vi "Delete Service.vi"(8 "error in (no error)":errorcluster, 10 "Service Name":string[][](array[string]), 11 "Manejo Turnos in":refnum<class "Manejo Turnos.lvclass">) -> (0 "error out":errorcluster, 3 "Manejo Turnos out":refnum<class "Manejo Turnos.lvclass">)   [LabVIEW 2020, in "Manejo Turnos.lvlib" / "Manejo Turnos.lvclass"]
uses:
  Manejo Turnos.lvclass
  C:/Program Files (x86)/National Instruments/LabVIEW 2020/vi.lib/ActorFramework/Actor/Actor.lvclass
  <vilib>/ActorFramework/Actor/Actor.lvclass/Actor.ctl
  <vilib>/ActorFramework/Message Enqueuer/Message Enqueuer.lvclass/Message Enqueuer.ctl
  Manejo Turnos.lvclass/Manejo Turnos.ctl
  <vilib>/ActorFramework/Message Enqueuer/Init from Existing Queue.vi
  <vilib>/ActorFramework/Message Enqueuer/Enqueue.vi
  Manejo Turnos Messages/Delete Services Table Msg/Delete Services Table Msg.lvclass
  C:/Program Files (x86)/National Instruments/LabVIEW 2020/vi.lib/ActorFramework/Message/Message.lvclass
  <vilib>/ActorFramework/Message Priority Queue/Priority Enqueue.vi
  <vilib>/ActorFramework/Message Enqueuer/Message Enqueuer.lvclass
  <vilib>/ActorFramework/Actor/Actor.lvclass
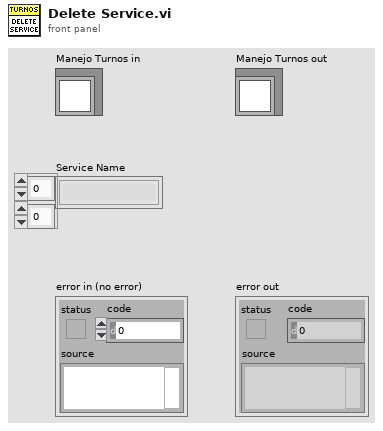
[diagram p1: front panel]
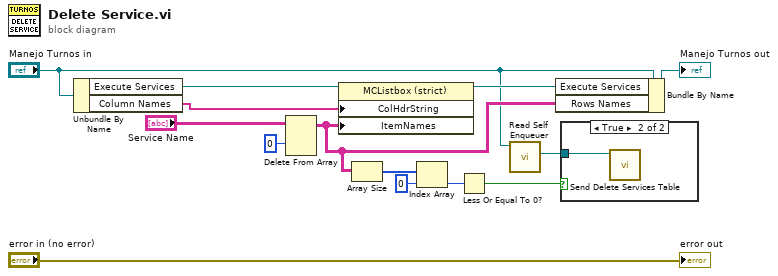
[diagram p0: block diagram]
diagram:
  n1 = Unbundle By Name("Manejo Turnos in") -> ("Execute Services"=w11:refnum<vi>, "Column Names"=w10:string[])
  n2 = Delete From Array(array="Service Name", index (row)=0) -> (array with subset deleted=w7:string[][])  [unwired: 2 in, 1 out]
  n3 = property class="MCListbox (strict)"(reference=w11, "ColHdrString"=w10, "ItemNames"=w7) -> (reference out=w12:refnum<vi>)  [unwired: 1 in, 1 out]
  n4 = Array Size(array=w7) -> (size(s)=w6:i32[])
  n5 = Index Array(array=w6, index=0) -> (element=w4:i32)
  n6 = Less Or Equal To 0?(x=w4) -> (x <= 0?=w3:bool)
  n7 = call <vilib>:"Read Self Enqueuer.vi"("Actor"="Manejo Turnos in") -> ("Self Enqueuer"=w1:refnum<class "Message Enqueuer.lvclass">)  [unwired: 10 in]
  n8 = Bundle By Name(cluster="Manejo Turnos in", "Execute Services"=w12, "Rows Names"=w7) -> (→"Manejo Turnos out":refnum<class "Manejo Turnos.lvclass">)
  n9 = case shown="True" w3 {
    tunnel: w1 -> [_ w15]
    frame False {
    }
    frame True {
      n10 = call "Send Delete Services Table.vi"("Message Enqueuer"=w15) -> ()  [unwired: 9 in, 2 out]
    }
  }
  "error out" <- "error in (no error)"
